vi "xycircle.vi"(9 "new picture in":picture, 10 "y":dbl, 11 "x":dbl) -> (3 "new picture out":picture)   [LabVIEW 2016]
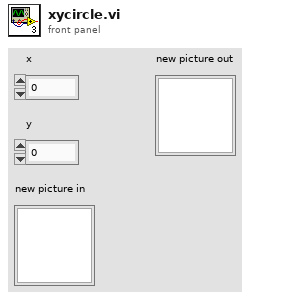
[diagram p1: front panel]
types:
  T1 = cluster{"Width":u16, "Style":enum32{"Solid", "Dash", "Dot", "DashDot", "DashDotDot"}}
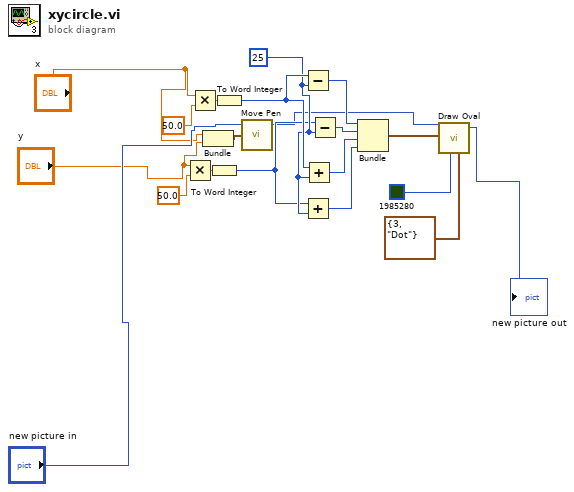
[diagram p0: block diagram]
diagram:
  w10 = i16 25 ("Waypoint \nSize")
  n1 = Multiply(x="y", y=50.0) -> (x*y=w9:dbl)
  n2 = Multiply(x="x", y=50.0) -> (x*y=w12:dbl)
  n3 = Bundle("x"="x", "y"="y") -> (w3:cluster{"x":dbl, "y":dbl})  [unwired: 1 in]
  n4 = To Word Integer(number=w9) -> (16bit integer=w7:i16)
  n5 = To Word Integer(number=w12) -> (16bit integer=w11:i16)
  n6 = call <vilib>:"Move Pen.vi"("new position"=w3, "picture"="new picture in") -> ("new picture"=w2:picture)  [unwired: 3 in]
  n7 = Subtract(x=w11, y=w10) -> (x-y=w17:i16)
  n8 = Add(x=w7, y=w10) -> (x+y=w14:i16)
  n9 = Add(x=w11, y=w10) -> (x+y=w15:i16)
  n10 = Subtract(x=w7, y=w10) -> (x-y=w16:i16)
  n11 = Bundle(w17, w16, w15, w14) -> (w5:cluster{i16, i16, i16, i16})  [unwired: 1 in]
  n12 = call <vilib>:"Draw Oval.vi"("picture"=w2, "rect"=w5, "color(black)"=u32 1985280, "pen"=T1 {"Width"=3, "Style"=enum."Dot"}) -> ("new picture"=→"new picture out":picture)  [unwired: 5 in]
